vi "Operate.vi"(8 "Error_In":errorcluster, 11 "Subtraction_In":refnum<class "Subtraction.lvclass">) -> (0 "Error_Out":errorcluster, 3 "Subtraction_Out":refnum<class "Subtraction.lvclass">)   [LabVIEW 2021, in "Subtraction.lvclass"]
doc: "Used to do Subtraction operation by over riding"
uses:
  Subtraction.lvclass
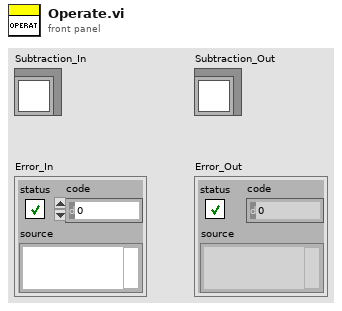
[diagram p1: front panel]
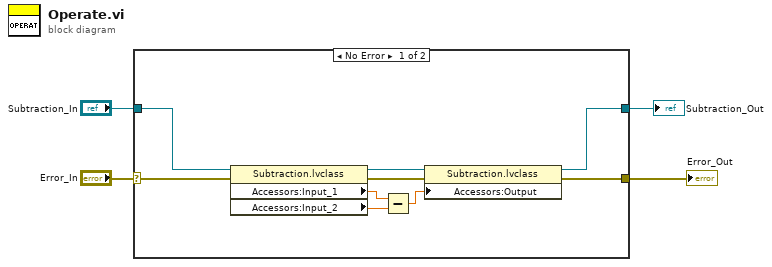
[diagram p0: block diagram]
diagram:
  n1 = case shown="No Error" "Error_In" {
    selector: "Error_In" -> [w13 w15]
    tunnel: [w11 w15] -> w3
    tunnel: [w9 w14] -> w1
    tunnel: "Subtraction_In" -> [w8 w14]
    frame No Error {
      n2 = property class="Subtraction.lvclass"(reference=w8, error in=w13) -> (reference out=w10:refnum<class "Subtraction.lvclass">, error out=w12:errorcluster, "Accessors:Input_1"=w7:dbl, "Accessors:Input_2"=w6:dbl)
      n3 = Subtract(x=w7, y=w6) -> (x-y=w5:dbl)
      n4 = property class="Subtraction.lvclass"(reference=w10, error in=w12, "Accessors:Output"=w5) -> (reference out=w9:refnum<class "Subtraction.lvclass">, error out=w11:errorcluster)
    }
    frame Error {
    }
  }
  "Subtraction_Out" <- w1
  "Error_Out" <- w3
